vi "Auto Align.vi"(4 "vision_deadzone":dbl, 5 "Vision PID":T9={"proportional gain (Kc)"=1.0, "integral time (Ti, min)"=0.01, "derivative time (Td, min)"=0.0} {"derivative time (Td, min)" format="%.3f"; "integral time (Ti, min)" format="%.3f"; "proportional gain (Kc)" format="%.3f"}, 6 "normalized coords":T1, 7 "fl_drive":T4, 8 "rr_drive":T4, 9 "rl_drive":T4, 10 "navX Device":T2 {"Interface"."Update Rate (4Hz-100Hz)" min=4 max=60 step=1}, 11 "fr_drive":T4) -> (3 "Finished":bool)   [LabVIEW 2018]
uses:
  <vilib>/Rock Robotics/WPI/MotorControl/WPI_MotorControlDeviceRef.ctl
  <vilib>/Rock Robotics/WPI/MotorControl/WPI_MotorControlType.ctl
  <vilib>/Rock Robotics/SystemInterfaces/DIO/FPGA_DIOPWMChannel.ctl
  <vilib>/Rock Robotics/WPI/PWM/WPI_PWMDeadband.ctl
  <vilib>/Rock Robotics/SystemInterfaces/DIO/FPGA_DIOChannel.ctl
  FIRST-3958-Controls-Library/NavX/navX Library v2/TypeDefs/Z900_navX_DeviceTypeDef.ctl
  FIRST-3958-Controls-Library/NavX/navX Library v2/TypeDefs/Z900_navX_ProtocolTypeDef.ctl
  FIRST-3958-Controls-Library/NavX/navX Library v2/TypeDefs/Z900_navX_NotifyPacketTypeDef.ctl
  FIRST-3958-Controls-Library/NavX/navX Library v2/TypeDefs/Z900_navX_ActionTypeDef.ctl
  <vilib>/addons/control/pid/pid.llb/PID (DBL).vi
  <vilib>/addons/control/pid/NI_PID_pid.lvlib
  FIRST-3958-Controls-Library/NavX/navX Library v2/navX Library v2.lvlib
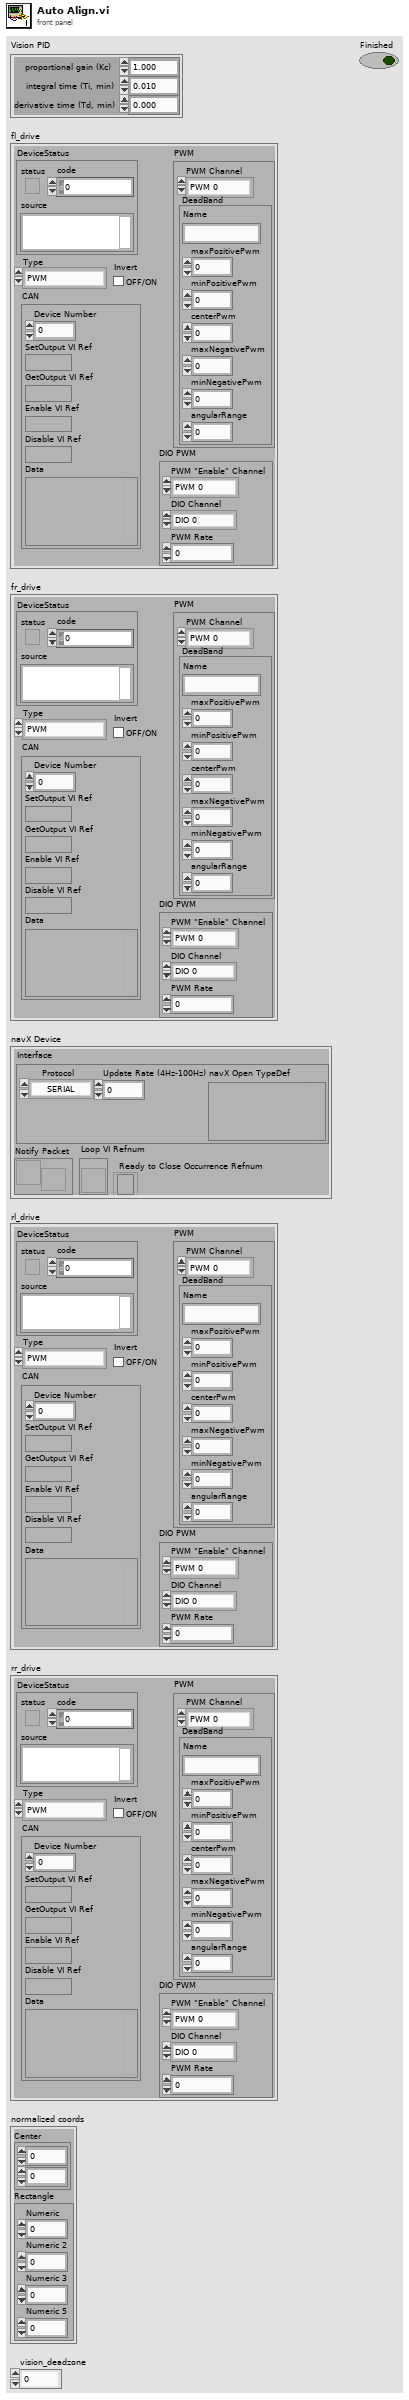
[diagram p1: front panel]
types:
  T1 = cluster{"Center":cluster{dbl, dbl}, "Rectangle":cluster{"Numeric":dbl, "Numeric 2":dbl, "Numeric 3":dbl, "Numeric 5":dbl}}
  T2 = typedef "navX Library v2.lvlib/Z900_navX_DeviceTypeDef.ctl" = cluster{"Interface":cluster{"Protocol":T3, "Update Rate (4Hz-100Hz)":u8, "navX Open TypeDef":variant}, "Notify Packet":refnum<notifier>, "Loop VI Refnum":refnum<vi>, "Ready to Close Occurrence Refnum":refnum<k4>}
  T3 = typedef "navX Library v2.lvlib/Z900_navX_ProtocolTypeDef.ctl" = enum16{"SERIAL", "I2C", "SPI"}
  T4 = typedef "WPI_MotorControlDeviceRef.ctl" = cluster{"DeviceStatus":errorcluster, "Type":T5, "PWM":cluster{"PWM Channel":T6, "DeadBand":T7}, "CAN":cluster{"Device Number":u8, "SetOutput VI Ref":variant, "GetOutput VI Ref":variant, "Enable VI Ref":variant, "Disable VI Ref":variant, "Data":variant}, "Invert":bool, "DIO PWM":cluster{"PWM \"Enable\" Channel":T6, "DIOChannel":T8, "PWM Rate":dbl}}
  T5 = typedef "WPI_MotorControlType.ctl" = enum16{"PWM", "CAN", "DIO PWM"}
  T6 = typedef "FPGA_DIOPWMChannel.ctl" = enum8{"PWM 0", "PWM 1", "PWM 2", "PWM 3", "PWM 4", "PWM 5", "PWM 6", "PWM 7", "PWM 8", "PWM 9", "PWM MXP 0", "PWM MXP 1", "PWM MXP 2", "PWM MXP 3", "PWM MXP 4", "PWM MXP 5", "PWM MXP 6", "PWM MXP 7", "PWM MXP 8", "PWM MXP 9", "Invalid"}
  T7 = typedef "WPI_PWMDeadband.ctl" = cluster{"Name":string, "maxPositivePwm":i32, "minPositivePwm":i32, "centerPwm":i32, "maxNegativePwm":i32, "minNegativePwm":i32, "angularRange":u16}
  T8 = typedef "FPGA_DIOChannel.ctl" = enum8{"DIO 0", "DIO 1", "DIO 2", "DIO 3", "DIO 4", "DIO 5", "DIO 6", "DIO 7", "DIO 8", "DIO 9", "DIO MXP 0", "DIO MXP 1", "DIO MXP 2", "DIO MXP 3", "DIO MXP 4", "DIO MXP 5", "DIO MXP 6", "DIO MXP 7", "DIO MXP 8", "DIO MXP 9", "DIO MXP 10", "DIO MXP 11", "DIO MXP 12", "DIO MXP 13", "DIO MXP 14", "DIO MXP 15", "SPI Port CS1", "SPI Port CS2", "SPI Port CS3", "SPI Port MISO", "SPI Port MOSI", "Invalid"}
  T9 = cluster{"proportional gain (Kc)":dbl, "integral time (Ti, min)":dbl, "derivative time (Td, min)":dbl}
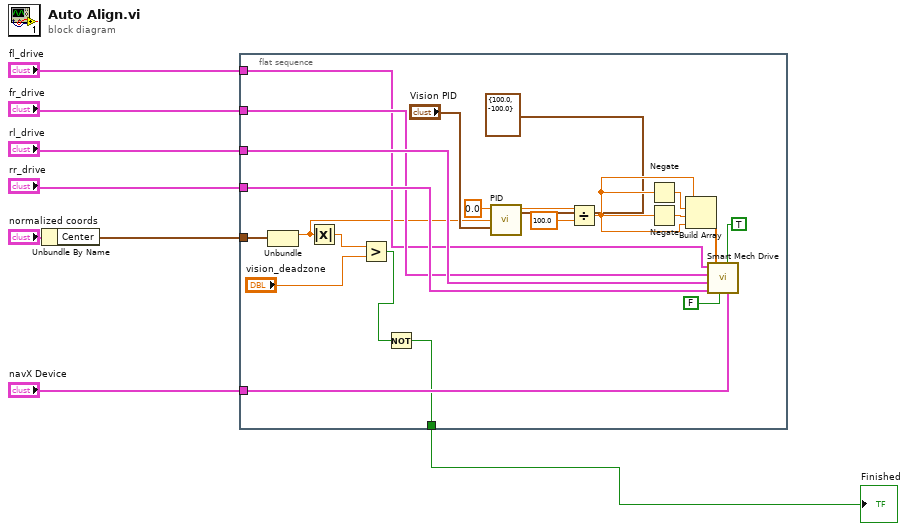
[diagram p0: block diagram]
diagram:
  n1 = Unbundle By Name("normalized coords") -> ("Center"=w2:cluster{dbl, dbl})
  n2 = flat-sequence {
    tunnel: "rr_drive" -> [w30]
    tunnel: "rl_drive" -> [w29]
    tunnel: "fr_drive" -> [w28]
    tunnel: "fl_drive" -> [w27]
    tunnel: "navX Device" -> [w26]
    tunnel: [w13] -> w3
    tunnel: w2 -> [w9]
    frame #0 {
      n3 = Unbundle(w9) -> (w15:dbl)  [unwired: 1 out]
      n4 = Absolute Value(x=w15) -> (abs(x)=w11:dbl)
      n5 = Greater?(x=w11, y="vision_deadzone") -> (0:w12:bool)
      n6 = Not(x=w12) -> (.not. x?=w13:bool)
      n7 = call-poly <vilib>:"PID.vi"("output range"=cluster{"output high":dbl, "output low":dbl} {"output high"=100.0, "output low"=-100.0}, "PID gains"="Vision PID", "process variable"=w15, "setpoint"=0.0) -> ("output"=w18:dbl)  [unwired: 6 in, 1 out]
      n8 = Divide(x=w18, y=100.0) -> (x/y=w22:dbl)
      n9 = Negate(x=w22) -> (-x=w21:dbl)
      n10 = Negate(x=w22) -> (-x=w20:dbl)
      n11 = Build Array(w22, w21, w20, w22) -> (w23:dbl[])
      n12 = call "Smart Mech Drive.vi"("navX Device"=w26, "rotation lock"=TRUE, "smart_drive"=FALSE, "motor values"=w23, "rr_motor"=w30, "rl_motor"=w29, "fr_motor"=w28, "fl_motor"=w27) -> ()  [unwired: 4 out]
    }
  }
  "Finished" <- w3
